vi "Column.vi"(7 "Blob?":bool, 8 "error in (no error)":errorcluster, 9 "iCol":i32, 10 "query return type":string, 11 "para0":u64) -> (0 "error out":errorcluster, 2 "function return":string, 3 "para0 out":u64)   [LabVIEW 2020, in "sqlite3.lvlib"]
uses:
  sqlite3.lvlib
  sqlite/subvi/Error Converter (ErrCode or Status).vi
  sqlite/VIs/errstr.vi
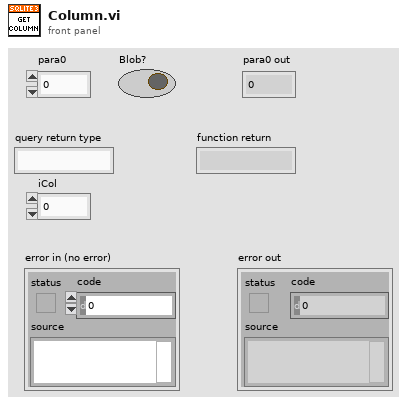
[diagram p1: front panel]
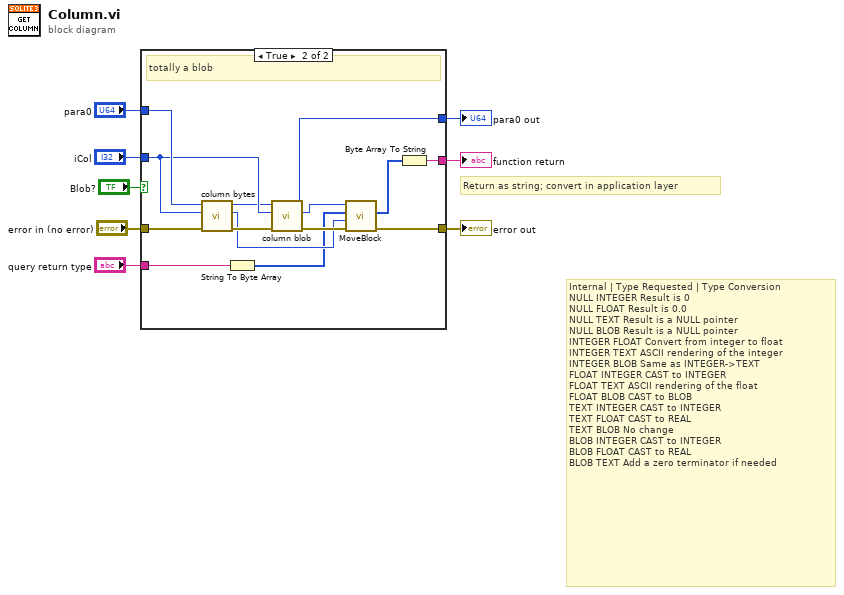
[diagram p0: block diagram]
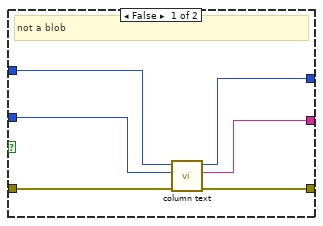
[diagram p2: hidden frame]
diagram:
  # "Return as string; convert in application layer"
  # "Internal | Type\tRequested | Type\tConversion\nNULL\tINTEGER\tResult is 0\nNULL\tFLOAT\tResult is 0.0\nNULL\tTEXT\tResult is a NULL pointer\nNULL\tBLOB\tResult is a NULL pointer\nINTEGER\tFLOAT\tConvert from integer to float\nINTEGER\tTEXT\tASCII rendering of the integer\nINTEGER\tBLOB\tSame as INTEGER->TEXT\nFLOAT\tINTEGER\tCAST to INTEGER\nFLOAT\tTEXT\tASCII rendering of the float\nFLOAT\tBLOB\tCAST to BLOB\nTEXT\tINTEGER\tCAST to INTEGER\nTEXT\tFLOAT\tCAST to REAL\nTEXT\tBLOB\tNo change\nBLOB\tINTEGER\tCAST to INTEGER\nBLOB\tFLOAT\tCAST to REAL\nBLOB\tTEXT\tAdd a zero terminator if needed"
  n1 = case shown="True" "Blob?" {
    tunnel: "query return type" -> [_ w18]
    tunnel: "error in (no error)" -> [w14 w28]
    tunnel: [w13 w25] -> w6
    tunnel: "para0" -> [w12 w27]
    tunnel: "iCol" -> [w11 w26]
    tunnel: [w10 w15] -> w3
    tunnel: [w9 w24] -> w2
    frame False {
      # "not a blob"
      n2 = call "column text.vi"("error in (no error)"=w14, "iCol"=w11, "para0"=w12) -> ("error out"=w13:errorcluster, "function return"=w10:string, "para0 out"=w9:u64)  [unwired: 6 in]
    }
    frame True {
      # "totally a blob"
      n3 = call "column bytes.vi"("error in (no error)"=w28, "iCol"=w26, "para0"=w27) -> ("error out"=w23:errorcluster, "column_bytes"=w20:i32, "para0 out"=w19:u64)  [unwired: 6 in]
      n4 = String To Byte Array(string=w18) -> (unsigned byte array=w17:u8[])
      n5 = call "column blob.vi"("error in (no error)"=w23, "iCol"=w26, "para0"=w19) -> ("error out"=w22:errorcluster, "function return"=w21:u64, "para0 out"=w24:u64)  [unwired: 6 in]
      n6 = call "MoveBlock.vi"("error in (no error)"=w22, "size"=w20, "destination (type)"=w17, "Address (pointer)"=w21) -> ("error out"=w25:errorcluster, "Value"=w16:u8[])  [unwired: 6 in]
      n7 = Byte Array To String(unsigned byte array=w16) -> (string=w15:string)
    }
  }
  "function return" <- w3
  "para0 out" <- w2
  "error out" <- w6
